vi "GetFrame.vi"(8 "error in (no error)":errorcluster, 10 "Image In":T1, 11 "Inovance_Camera in":refnum<class "Inovance_Camera.lvclass">) -> (0 "error out":errorcluster, 3 "Inovance_Camera out":refnum<class "Inovance_Camera.lvclass">)   [LabVIEW 2023, in "Inovance_Camera.lvlib" / "Inovance_Camera.lvclass"]
uses:
  Inovance_Camera.lvclass
  C:/Program Files/National Instruments/LabVIEW 2023/vi.lib/ActorFramework/Actor/Actor.lvclass
  <vilib>/vision/Image Controls.llb/IMAQ Image.ctl
  <vilib>/userDefined/High Color/IMAQdx.ctl
  <vilib>/ActorFramework/Actor/Actor.lvclass/Actor.ctl
  Inovance_Camera.lvclass/Inovance_Camera.ctl
  Interfaces/AbstractInstrumentClasses/Cameras_LV/CameraComm Messages/Frame Ready Msg/Frame Ready Msg.lvclass/Frame Ready Msg.ctl
  <vilib>/ActorFramework/Message Enqueuer/Message Enqueuer.lvclass/Message Enqueuer.ctl
  <vilib>/ActorFramework/Message Enqueuer/Enqueue.vi
  Interfaces/AbstractInstrumentClasses/Cameras_LV/CameraComm Messages/Frame Ready Msg/Frame Ready Msg.lvclass
  C:/Program Files/National Instruments/LabVIEW 2023/vi.lib/ActorFramework/Message/Message.lvclass
  <vilib>/ActorFramework/Message Priority Queue/Priority Enqueue.vi
  <vilib>/vision/driver/NI_Vision_Acquisition_Software.lvlib
  <vilib>/ActorFramework/Actor/Actor.lvclass
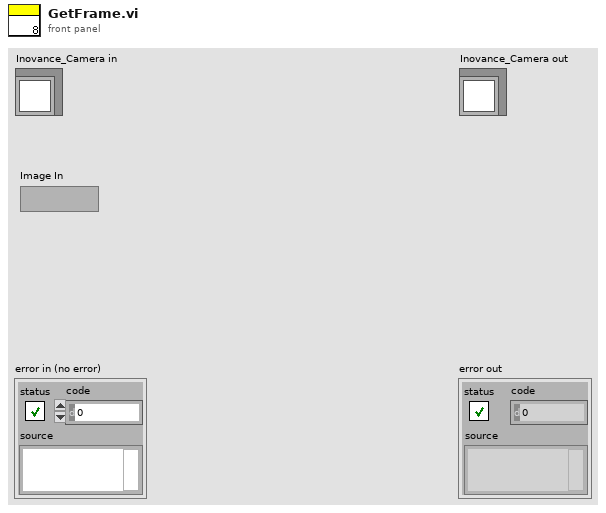
[diagram p1: front panel]
types:
  T1 = typedef "IMAQ Image.ctl" = refnum<image>
  T2 = typedef "IMAQdx.ctl" = refnum<k21>
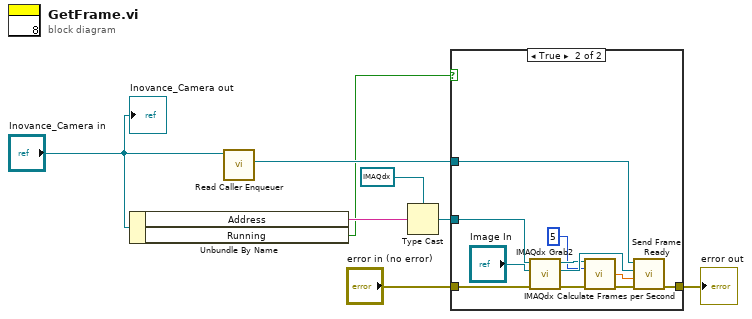
[diagram p0: block diagram]
diagram:
  n1 = Unbundle By Name("Inovance_Camera in") -> ("Address"=w3:string, "Running"=w2:bool)
  n2 = call <vilib>:"Read Caller Enqueuer.vi"("Actor"="Inovance_Camera in") -> ("Caller Enqueuer"=w8:refnum<class "Message Enqueuer.lvclass">)  [unwired: 10 in]
  n3 = Type Cast(type=T2 refnum ("Inovance Address"), x=w3) -> (*(type *) &x=w4:T2)
  n4 = case shown="True" w2 {
    tunnel: w8 -> [_ w19]
    tunnel: [w9 w17] -> w7
    tunnel: w4 -> [_ w16]
    tunnel: "error in (no error)" -> [w9 w10]
    frame False {
    }
    frame True {
      n5 = call <vilib>:"IMAQdx Grab2.vi"("error in"=w10, "Image In"="Image In", "Session In"=w16) -> ("error out"=w15:errorcluster, "Image Out"=w18:T1, "Session Out"=w13:T2)  [unwired: 5 in, 1 out]
      n6 = call <vilib>:"IMAQdx Calculate Frames per Second.vi"("Session In"=w13, "Buffer Number"=u32 5, "error in (no error)"=w15) -> ("Processed Frames per Second"=w11:dbl, "error out"=w14:errorcluster)  [unwired: 6 in, 5 out]
      n7 = call "Send Frame Ready.vi"("error in (no error)"=w14, "Processed Frames per Second"=w11, "Image In"=w18, "Message Enqueuer"=w19) -> ("error out"=w17:errorcluster)  [unwired: 6 in, 1 out]
    }
  }
  "error out" <- w7
  "Inovance_Camera out" <- "Inovance_Camera in"
